vi "Cleanup Wire on Terminal.vi"(5 "Remove Loose Ends":bool, 7 "Clean Up wire":bool=TRUE, 8 "error in":errorcluster, 10 "Wire In":refnum<vi>, 11 "Terminal in":refnum<vi>) -> (0 "error out":errorcluster, 2 "Wire out":refnum<vi>, 3 "Terminal Out":refnum<vi>)   [LabVIEW 2023]
doc: "Given a terminal OR wire reference, clean up wire. Output terminals may not be valid depending on if there was a wire and which input terminal was wired."
panel:
  # "OR"
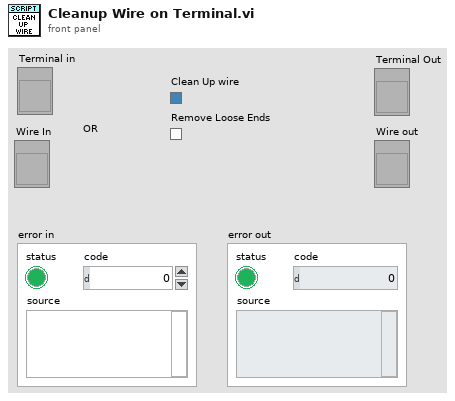
[diagram p1: front panel]
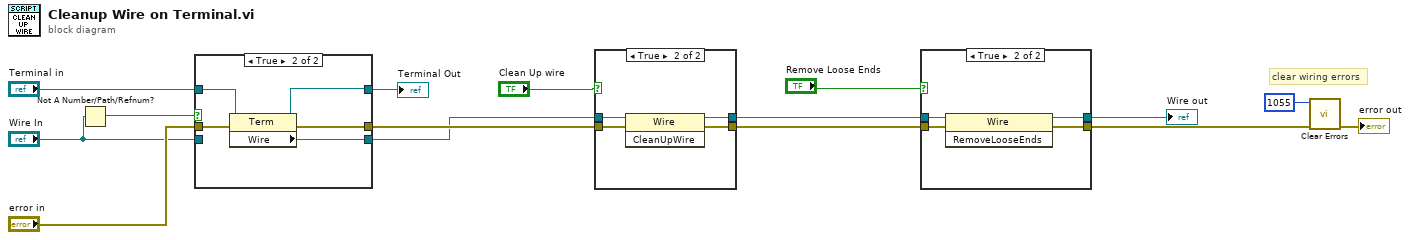
[diagram p0: block diagram]
diagram:
  # "clear wiring errors"
  n1 = Not A Number/Path/Refnum?(number/path/refnum="Wire In") -> (NaN/Path/Refnum?=w8:bool)
  n2 = case shown="True" w8 {
    tunnel: [w17 w23] -> w15
    tunnel: "error in" -> [w17 w22]
    tunnel: [w18 w21] -> w11
    tunnel: "Terminal in" -> [w16 w20]
    tunnel: "Wire In" -> [w18 _]
    tunnel: [w16 w19] -> w7
    frame False {
    }
    frame True {
      n3 = property class="Term"(reference=w20, error in=w22) -> (reference out=w19:refnum<vi>, error out=w23:errorcluster, "Wire"=w21:refnum<vi>)
    }
  }
  "Terminal Out" <- w7
  n4 = case shown="True" "Clean Up wire" {
    tunnel: [w25 w29] -> w5
    tunnel: [w24 w28] -> w4
    tunnel: w15 -> [w24 w27]
    tunnel: w11 -> [w25 w26]
    frame False {
    }
    frame True {
      n5 = invoke class="Wire" method="CleanUpWire"(reference=w26, error in=w27) -> (reference out=w29:refnum<vi>, error out=w28:errorcluster)  [unwired: 1 in, 1 out]
    }
  }
  n6 = case shown="True" "Remove Loose Ends" {
    tunnel: [w31 w33] -> w3
    tunnel: [w30 w32] -> w2
    tunnel: w4 -> [w30 w34]
    tunnel: w5 -> [w31 w35]
    frame False {
    }
    frame True {
      n7 = invoke class="Wire" method="RemoveLooseEnds"(reference=w35, error in=w34) -> (reference out=w33:refnum<vi>, error out=w32:errorcluster)  [unwired: 1 in, 1 out]
    }
  }
  "Wire out" <- w3
  n8 = call <vilib>:"Clear Errors.vi"("error in (no error)"=w2, "specific error code to clear (0: all)"=1055) -> ("error out"=→"error out":errorcluster)  [unwired: 4 in, 1 out]
